vi "initialise.vi"(8 "error in (no error)":errorcluster, 11 "scriptFileName":string) -> (0 "error out":errorcluster, 3 "function return":i32)   [LabVIEW 2011, in "GlazLib.lvlib"]
doc: "DECLSPEC int CDECL initialiseSession(const char* scriptFileName);"
uses:
  GlazLib.lvlib
  <userlib>/GlazLabView/GlazLib.dll
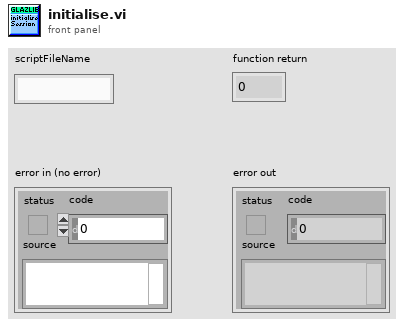
[diagram p1: front panel]
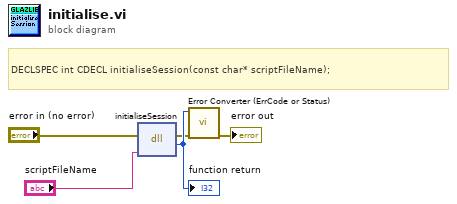
[diagram p0: block diagram]
diagram:
  # "DECLSPEC int CDECL initialiseSession(const char* scriptFileName);"
  n1 = dll-call lib="C:/Program Files (x86)/National Instruments/LabVIEW 2015/user.lib/GlazLabView/GlazLib.*" fn="initialiseSession"(error in="error in (no error)", "scriptFileName"="scriptFileName") -> (error out=w2:errorcluster, w5:i32)  [unwired: 3 in, 1 out]
  "function return" <- w5
  n2 = call "Error Converter (ErrCode or Status).vi"("error in (no error)"=w2, "error code"=w5) -> ("error out"=→"error out":errorcluster)  [unwired: 9 in]
